vi "MCListbox - Reset Color.vi"(11 "MulticolumnListbox in":refnum<vi>) -> (3 "MulticolumnListbox out":refnum<vi>)   [LabVIEW 2013]
uses:
  <vilib>/Utility/miscctls.llb/LVRowAndColumnTypeDef.ctl
  Controls/MCListbox - Enum.ctl
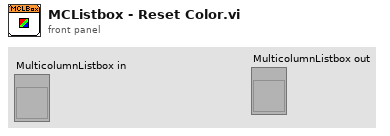
[diagram p1: front panel]
types:
  T1 = typedef "MCListbox - Enum.ctl" = enum16{"Initial (KD?)", "Initial Text", "B4 <Return>", "Now", "Max row count", "Mandatory Fields", "Data Type", "Stored Row, Col, Color"}
  T2 = typedef "LVRowAndColumnTypeDef.ctl" = cluster{"Row":i32, "Column":i32}
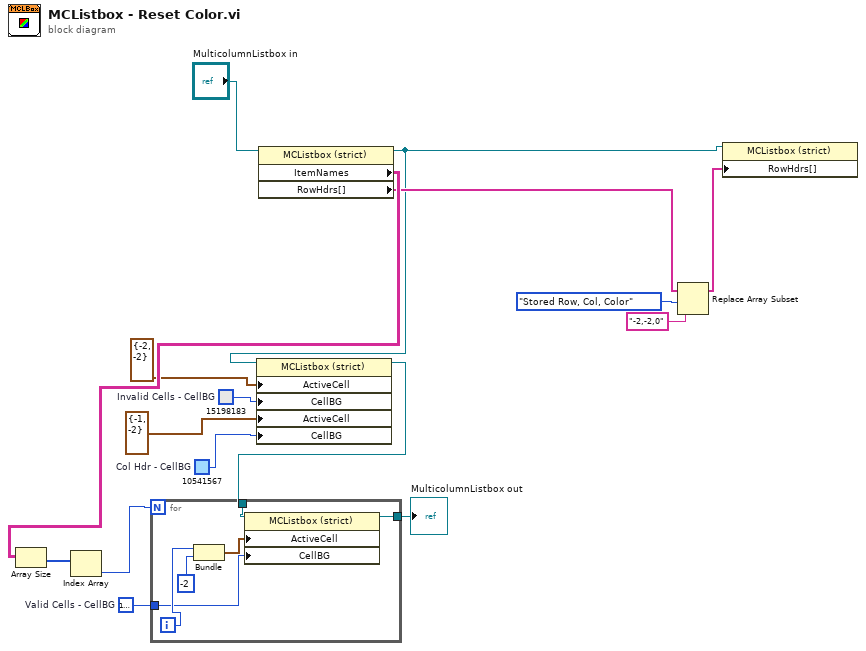
[diagram p0: block diagram]
diagram:
  w14 = u32 16777226  # Valid Cells - CellBG
  w10 = u32 10541567  # Col Hdr - CellBG
  w7 = u32 15198183  # Invalid Cells - CellBG
  n1 = property on="Property Node" class="MCListbox (strict)"(reference="MulticolumnListbox in") -> (reference out=w2:refnum<vi>, "ItemNames"=w16:string[][], "RowHdrs[]"=w4:string[])  [unwired: 1 in, 1 out]
  n2 = Array Size(array=w16) -> (size(s)=w12:i32[])
  n3 = Index Array(array=w12) -> (element=w13:i32)  [unwired: 1 in]
  n4 = property on="Property Node" class="MCListbox (strict)"(reference=w2, "ActiveCell"=T2 {"Row"=-2, "Column"=-2} ("Active Cell:Active Cell"), "CellBG"=w7, "ActiveCell"=T2 {"Row"=-1, "Column"=-2} ("Active Cell:Active Cell"), "CellBG"=w10) -> (reference out=w11:refnum<vi>)  [unwired: 1 in, 1 out]
  n5 = for {
    N: w13 -> [_]
    tunnel: w11 -> [w22]
    tunnel: w14 -> [w18]
    tunnel: [w17] -> w6
    i -> [w21]
    n6 = Bundle(w21, -2) -> (w19:cluster{i32, i32})  [unwired: 1 in]
    n7 = property on="Property Node" class="MCListbox (strict)"(reference=w22, "ActiveCell"=w19, "CellBG"=w18) -> (reference out=w17:refnum<vi>)  [unwired: 1 in, 1 out]
  }
  "MulticolumnListbox out" <- w6
  n8 = Replace Array Subset(array=w4, new element="-2,-2,0" ("new element/subarray"), index=MCListbox_-_Enum."Stored Row, Col, Color" ("MCListbox Enum")) -> (w1:string[])
  n9 = property on="Property Node" class="MCListbox (strict)"(reference=w2, "RowHdrs[]"=w1) -> ()  [unwired: 1 in, 2 out]
